vi "Measure.vi"(8 "error in (no error)":errorcluster, 9 "measurement configuration":variant, 10 "measure call context in":refnum<class "Measure Call Context.lvclass">, 11 "measurement plugin in":refnum<class "CAN-LIN Frame Generator.lvclass">) -> (0 "error out":errorcluster, 1 "measurement results":variant, 2 "measure call context out":refnum<class "Measure Call Context.lvclass">, 3 "measurement plugin out":refnum<class "CAN-LIN Frame Generator.lvclass">)   [LabVIEW 2025, in "CAN-LIN Frame Generator.lvclass"]
uses:
  CAN-LIN Frame Generator.lvclass
  <vilib>/Plug-In SDKs/Measurements/Measure Call Context/Measure Call Context.lvclass
  Measurement Configuration.ctl
  CAN-LIN Frame Generator UI/Toggle.ctl
  CAN-LIN Frame Generator.lvclass/CAN-LIN Frame Generator.ctl
  OOB gRPC Server/OOB gRPC Server.lvlib
  OOB Data Transfer/OOB Data Transfer.lvlib
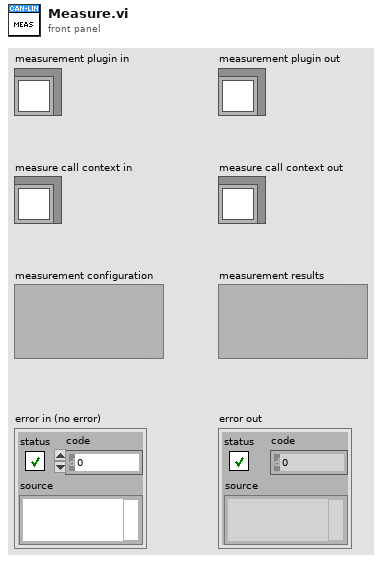
[diagram p1: front panel]
types:
  T1 = typedef "CAN-LIN Frame Generator.lvclass/Measurement Configuration.ctl" = cluster{"INTERFACE NAME CAN":refnum<k21>, "IO Mode CAN":enum32{"CAN", "CAN FD", "CAN FD + BRS"}, "FD ISO Mode CAN":enum32{"ISO", "Legacy ISO", "Non-ISO"}, "Termination CAN":T2, "Baudrate CAN":u32, "FD Baudrate CAN":u32, "INTERFACE NAME LIN":refnum<k21>, "Termination LIN":T2, "CAN interface":string, "LIN interface":string, "Network":string, "Baudrate LIN":u32}
  T2 = typedef "Toggle.ctl" = bool
  T3 = typedef "CAN-LIN Frame Generator.lvclass/Measurement Results.ctl" = cluster{"OOB gRPC Port":i32, "ID CAN":u32, "DLC CAN":u32, "SEND CAN":bool, "Payload CAN":u32[], "ID LIN":u32, "DLC LIN":u32, "SEND LIN":bool, "Payload LIN":u32[], "out_str":string}
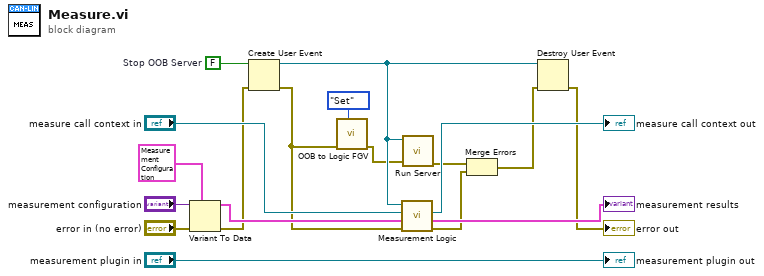
[diagram p0: block diagram]
diagram:
  w1 = FALSE  # Stop OOB Server
  n1 = Variant To Data(error in="error in (no error)", type=T1 {"INTERFACE NAME CAN"="Lorem ipsum dolor sit", "IO Mode CAN"=enum."CAN FD", "FD ISO Mode CAN"=enum."Non-ISO", "Termination CAN"=TRUE, "Baudrate CAN"=64, "FD Baudrate CAN"=64, "INTERFACE NAME LIN"="", "Termination LIN"=TRUE, "CAN interface"="", "LIN interface"="", "Network"="", "Baudrate LIN"=0} ("measurement configuration"), Variant="measurement configuration") -> (data=w11:T1, error out=w10:errorcluster)
  n2 = Create User Event(user event datatype=w1, error in=w10) -> (user event=w9:refnum<user-event>, error out=w4:errorcluster)
  n3 = call "OOB to Logic FGV.vi"("Op (Get)"=enum16{"Get", "Set"}."Set", "error in (no error)"=w4) -> ("error out"=w2:errorcluster)  [unwired: 8 in, 1 out]
  n4 = call "Measurement Logic.vi"("error in"=w4, "measurement configuration"=w11, "measure call context in"="measure call context in", "Stop OOB Server UE"=w9) -> ("error out"=w7:errorcluster, "measurement results"=→"measurement results":T3, "measure call context out"=→"measure call context out":refnum<class "Measure Call Context.lvclass">)  [unwired: 5 in]
  n5 = call "Run Server.vi"("error in (no error)"=w2, "Stop OOB Server UE"=w9) -> ("error out"=w6:errorcluster)  [unwired: 9 in]
  n6 = Merge Errors(w6, w7) -> (w5:errorcluster)
  n7 = Destroy User Event(user event=w9, error in=w5) -> (error out=→"error out":errorcluster)
  "measurement plugin out" <- "measurement plugin in"
